vi "Send Set Timer.vi"(7 "Message Priority (Normal)":T2=enum."Normal", 8 "error in (no error)":errorcluster, 9 "State":T1, 10 "Target time":dbl, 11 "Message Enqueuer":refnum<class "Message Enqueuer.lvclass">) -> (0 "error out":errorcluster, 3 "Message Enqueuer out":refnum<class "Message Enqueuer.lvclass">)   [LabVIEW 2019, in "ATM Controller.lvlib" / "Set Timer Msg.lvclass"]
doc: "This VI sends the message to an actor."
uses:
  Set Timer Msg.lvclass
  <vilib>/ActorFramework/Message Enqueuer/Message Enqueuer.lvclass
  <vilib>/ActorFramework/Message Enqueuer/Message Priority.ctl
  ATM Controller/State -Enum.ctl
  C:/Program Files (x86)/National Instruments/LabVIEW 2019/vi.lib/ActorFramework/Message/Message.lvclass
  Set Timer Msg.lvclass/Set Timer Msg.ctl
  <vilib>/ActorFramework/Message Enqueuer/Message Enqueuer.lvclass/Message Enqueuer.ctl
  <vilib>/ActorFramework/Message Priority Queue/Priority Enqueue.vi
  ATM Controller/ATM Controller.lvclass
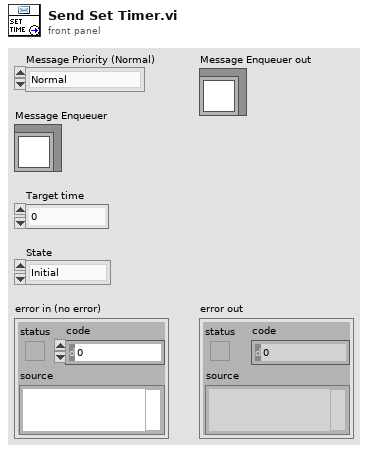
[diagram p1: front panel]
types:
  T1 = typedef "ATM Controller.lvlib/ATM Controller.lvclass/State -Enum.ctl" = enum16{"Initial", "Idle", "Login", "Balance Inquiry", "Deposit", "Withdrawal", "Fast Cash", "Terminate", "Inactivity Timeout"}
  T2 = typedef "Actor Framework.lvlib/Message Enqueuer.lvclass/Message Priority.ctl" = enum16{"Low", "Normal", "High"}
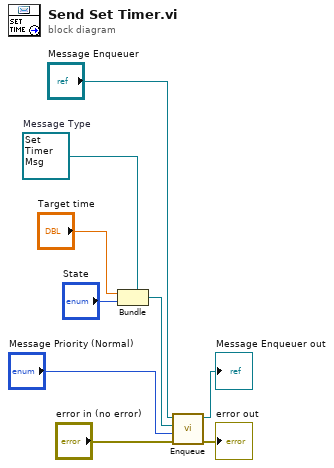
[diagram p0: block diagram]
diagram:
  w3 = refnum<class "Set Timer Msg.lvclass"> refnum  # Message Type
  n1 = Bundle(cluster=w3, "Target time", "State") -> (w4:refnum<class "Set Timer Msg.lvclass">)
  n2 = call <vilib>:"Enqueue.vi"("error in (no error)"="error in (no error)", "Message Priority (Normal)"="Message Priority (Normal)", "Message"=w4, "Message Enqueuer in"="Message Enqueuer") -> ("error out"=→"error out":errorcluster, "Message Enqueuer out"=→"Message Enqueuer out":refnum<class "Message Enqueuer.lvclass">)  [unwired: 6 in]
